vi "Find path stem.vi"() -> (0 "PASS/FAIL":bool, 1 "Path stem.":path)   [LabVIEW 2010]
panel:
  # "No inputs:"
  # "Outputs:"
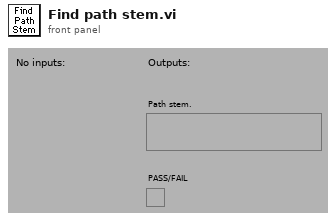
[diagram p1: front panel]
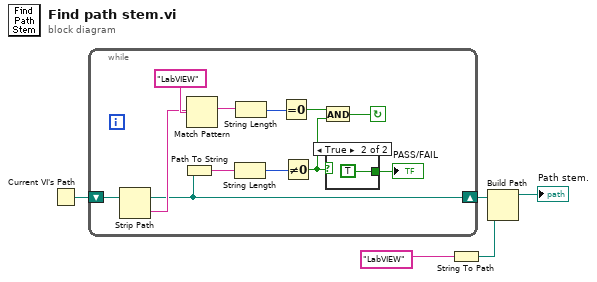
[diagram p0: block diagram]
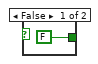
[diagram p2: hidden frame]
diagram:
  n1 = Current VI's Path() -> (path=w5:path)
  n2 = while {
    shift-left: w5 -> [w16]
    shift-right: [w11] -> w2
    stop <- w6 continue-if-true
    n3 = Strip Path(path=w16) -> (stripped path=w11:path, name=w15:string)
    n4 = Path To String(path=w11) -> (string=w13:string)
    n5 = Match Pattern(string=w15, regular expression="LabVIEW") -> (match substring=w14:string)  [unwired: 4 out]
    n6 = String Length(string=w13) -> (length=w12:i32)
    n7 = String Length(string=w14) -> (length=w9:i32)
    n8 = Equal To 0?(x=w9) -> (x = 0?=w8:bool)
    n9 = Not Equal To 0?(x=w12) -> (x != 0?=w7:bool)
    n10 = And(x=w8, y=w7) -> (x .and. y?=w6:bool)
    n11 = case shown="True" w7 {
      tunnel: [FALSE TRUE] -> w10
      frame False {
      }
      frame True {
      }
    }
    "PASS/FAIL" <- w10
  }
  n12 = String To Path(string="LabVIEW") -> (path=w3:path)
  n13 = Build Path(base path=w2, name or relative path=w3) -> (appended path=→"Path stem.":path)
